vi "set_ref_clus_MKS946.vi"(6 "cluster_ref":T1, 9 "PR2":dbl, 10 "PR1":dbl, 11 "status":bool) -> ()   [LabVIEW 2019]
uses:
  cluster_ref_MKS946.ctl
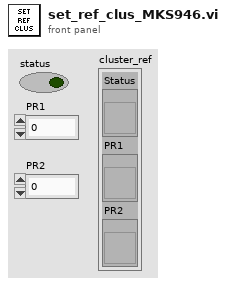
[diagram p1: front panel]
types:
  T1 = typedef "cluster_ref_MKS946.ctl" = cluster{"Status":refnum<vi>, "PR1":refnum<vi>, "PR2":refnum<vi>}
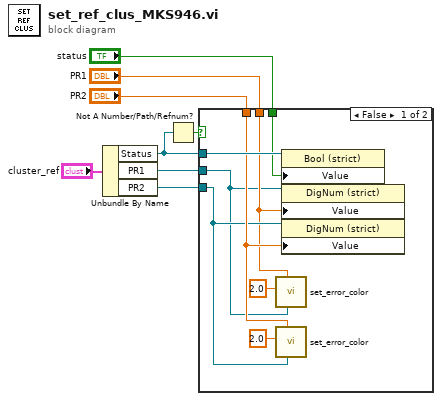
[diagram p0: block diagram]
diagram:
  n1 = Unbundle By Name("cluster_ref") -> ("Status"=w6:refnum<vi>, "PR1"=w5:refnum<vi>, "PR2"=w4:refnum<vi>)
  n2 = Not A Number/Path/Refnum?(number/path/refnum=w6) -> (NaN/Path/Refnum?=w7:bool)
  n3 = case shown="False" w7 {
    tunnel: w6 -> [w16 _]
    tunnel: w5 -> [w10 _]
    tunnel: w4 -> [w13 _]
    tunnel: "status" -> [w15 _]
    tunnel: "PR1" -> [w11 _]
    tunnel: "PR2" -> [w14 _]
    frame False {
      n4 = call "set_error_color.vi"("value_ref"=w10, "value"=w11, "hi"=2.0) -> ()  [unwired: 9 in]
      n5 = call "set_error_color.vi"("value_ref"=w13, "value"=w14, "hi"=2.0) -> ()  [unwired: 9 in]
      n6 = property class="Bool (strict)"(reference=w16, "Value"=w15) -> ()  [unwired: 1 in, 2 out]
      n7 = property class="DigNum (strict)"(reference=w10, "Value"=w11) -> ()  [unwired: 1 in, 2 out]
      n8 = property class="DigNum (strict)"(reference=w13, "Value"=w14) -> ()  [unwired: 1 in, 2 out]
    }
    frame True {
    }
  }
